vi "__Cloud List Menu Delete Handler.vi"(7 "FileManager Data":T1, 8 "error in (no error)":errorcluster) -> (0 "error out":errorcluster)   [LabVIEW 2011]
doc: "Handles the delete operation on the cloud list."
uses:
  __File manager Data type.ctl
  vi.lib/National Instruments/LabVIEW Interface for Amazon S3/LV Interface for Amazon S3.lvlib
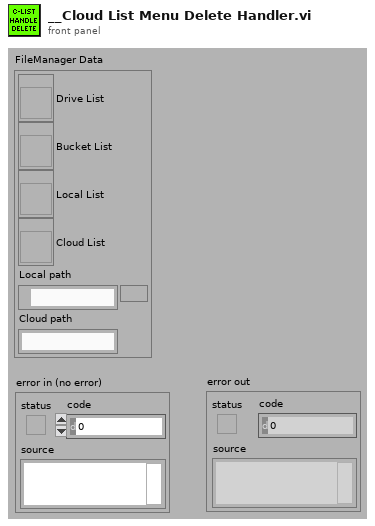
[diagram p1: front panel]
types:
  T1 = typedef "__File manager Data type.ctl" = cluster{"Drive List":refnum<vi>, "Bucket List":refnum<vi>, "Local List":refnum<vi>, "Cloud List":refnum<vi>, "Local path":path, "Cloud path":string}
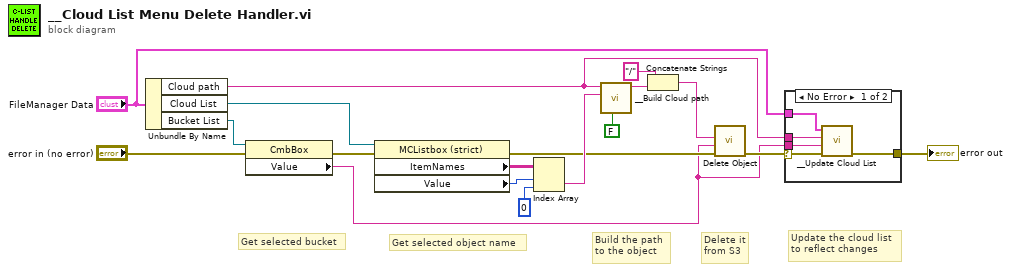
[diagram p0: block diagram]
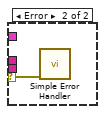
[diagram p2: hidden frame]
diagram:
  # "Update the cloud list\nto reflect changes"
  # "Delete it\nfrom S3"
  # "Build the path\nto the object"
  # "Get selected bucket"
  # "Get selected object name"
  n1 = Unbundle By Name("FileManager Data") -> ("Cloud path"=w2:string, "Cloud List"=w16:refnum<vi>, "Bucket List"=w18:refnum<vi>)
  n2 = property class="CmbBox"(reference=w18, error in="error in (no error)") -> (error out=w15:errorcluster, "Value"=w1:string)  [unwired: 1 out]
  n3 = property class="MCListbox (strict)"(reference=w16, error in=w15) -> (error out=w10:errorcluster, "ItemNames"=w14:string[][], "Value"=w13:i32)  [unwired: 1 out]
  n4 = Index Array(array=w14, index (row)=w13, index (col)=0 ("disabled index (col)")) -> (element=w11:string)
  n5 = call "__Build Cloud path.vi"("Folder?"=FALSE, "New Path element"=w11, "Current Cloud path"=w2) -> ("New Cloud path"=w8:string)  [unwired: 8 in]
  n6 = Concatenate Strings("/" ("string"), w8) -> (w6:string)
  n7 = call "Delete Object.vi"("error in (no error)"=w10, "Bucket"=w1, "Object path"=w6) -> ("error out"=w5:errorcluster)  [unwired: 7 in, 1 out]
  n8 = case shown="No Error" w5 {
    selector: w5 -> [w23 w24]
    tunnel: [w22 _] -> w4
    tunnel: "FileManager Data" -> [w21 _]
    tunnel: w2 -> [w20 _]
    tunnel: w1 -> [w19 _]
    frame No Error {
      n9 = call "__Update Cloud List.vi"("error in (no error)"=w23, "Bucket"=w19, "Path to list"=w20, "FileManager Ctl Refs in"=w21) -> ("error out"=w22:errorcluster)  [unwired: 6 in, 1 out]
    }
    frame Error {
      n10 = call <vilib>:"Simple Error Handler.vi"("error in (no error)"=w24) -> ()  [unwired: 4 in, 5 out]
    }
  }
  "error out" <- w4
